vi "Check File Existence.vi"(8 "error in (no error)":errorcluster, 11 "Config_Read in":refnum<class "Config_Read_BML.lvclass">) -> (0 "error out":errorcluster, 3 "Config_Read out":refnum<class "Config_Read_BML.lvclass">)   [LabVIEW 2018, in "Config_Read_BML.lvclass"]
uses:
  Config_Read_BML.lvclass
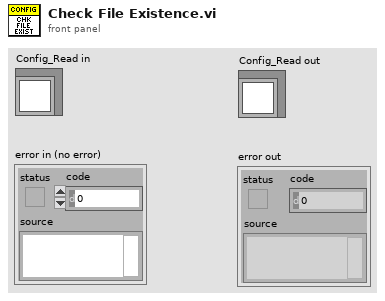
[diagram p1: front panel]
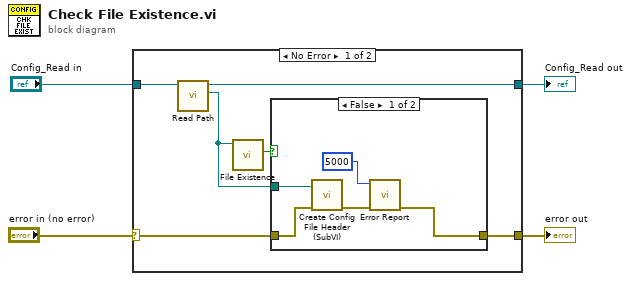
[diagram p0: block diagram]
diagram:
  n1 = case shown="No Error" "error in (no error)" {
    selector: "error in (no error)" -> [w7 w17]
    tunnel: [w8 w17] -> w3
    tunnel: [w9 w18] -> w1
    tunnel: "Config_Read in" -> [w10 w18]
    frame No Error {
      n2 = call-dynamic "Read Path.vi"("Config_Read in"=w10) -> ("Path"=w5:path, "Config_Read out"=w9:refnum<class "Config_Read_BML.lvclass">)  [unwired: 8 in, 1 out]
      n3 = call "File Existence"("file path"=w5) -> ("exists"=w6:bool)  [unwired: 9 in, 1 out]
      n4 = case shown="False" w6 {
        tunnel: w5 -> [w15 _]
        tunnel: [w12 w16] -> w8
        tunnel: w7 -> [w11 w16]
        frame False {
          n5 = call "Create Config File Header (SubVI).vi"("error in (no error)"=w11, "file path"=w15) -> ("error out"=w14:errorcluster)  [unwired: 8 in, 1 out]
          n6 = call "Error Report.vi"("error in (no error)"=w14, "Error Code"=i16 5000) -> ("error out"=w12:errorcluster)  [unwired: 9 in]
        }
        frame True {
        }
      }
    }
    frame Error {
    }
  }
  "error out" <- w3
  "Config_Read out" <- w1
